vi "wavelenght and intensity New.vi"(8 "Command":string, 10 "Number of Fiber":string, 11 "VISA resource name":string) -> (0 "LED":bool, 1 "LED COLOR":string, 2 "INTENSITY":i32, 3 "WAVELENGHT":dbl)   [LabVIEW 2023]
panel:
  out "number_LED":i32
  out "Blue":u8
  out "Green":u8
  out "Red":u8
  out "VISA resource name":refnum<visa-resource-name>="ASRL34::INSTR"
  out "OUTPUT":string
  # "NOTE: remember plug-in the LED Analyser\ncable before run this VI and to select the\nVISA resource name (port)"
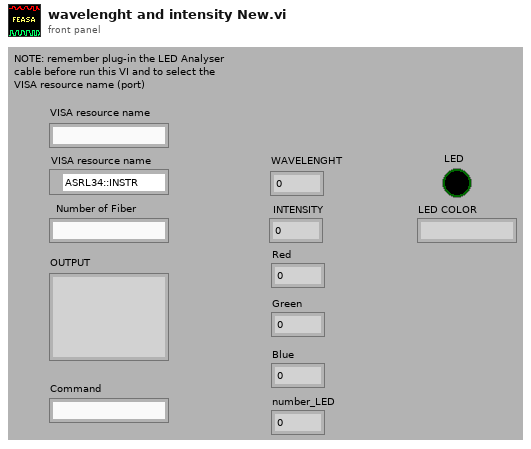
[diagram p1: front panel]
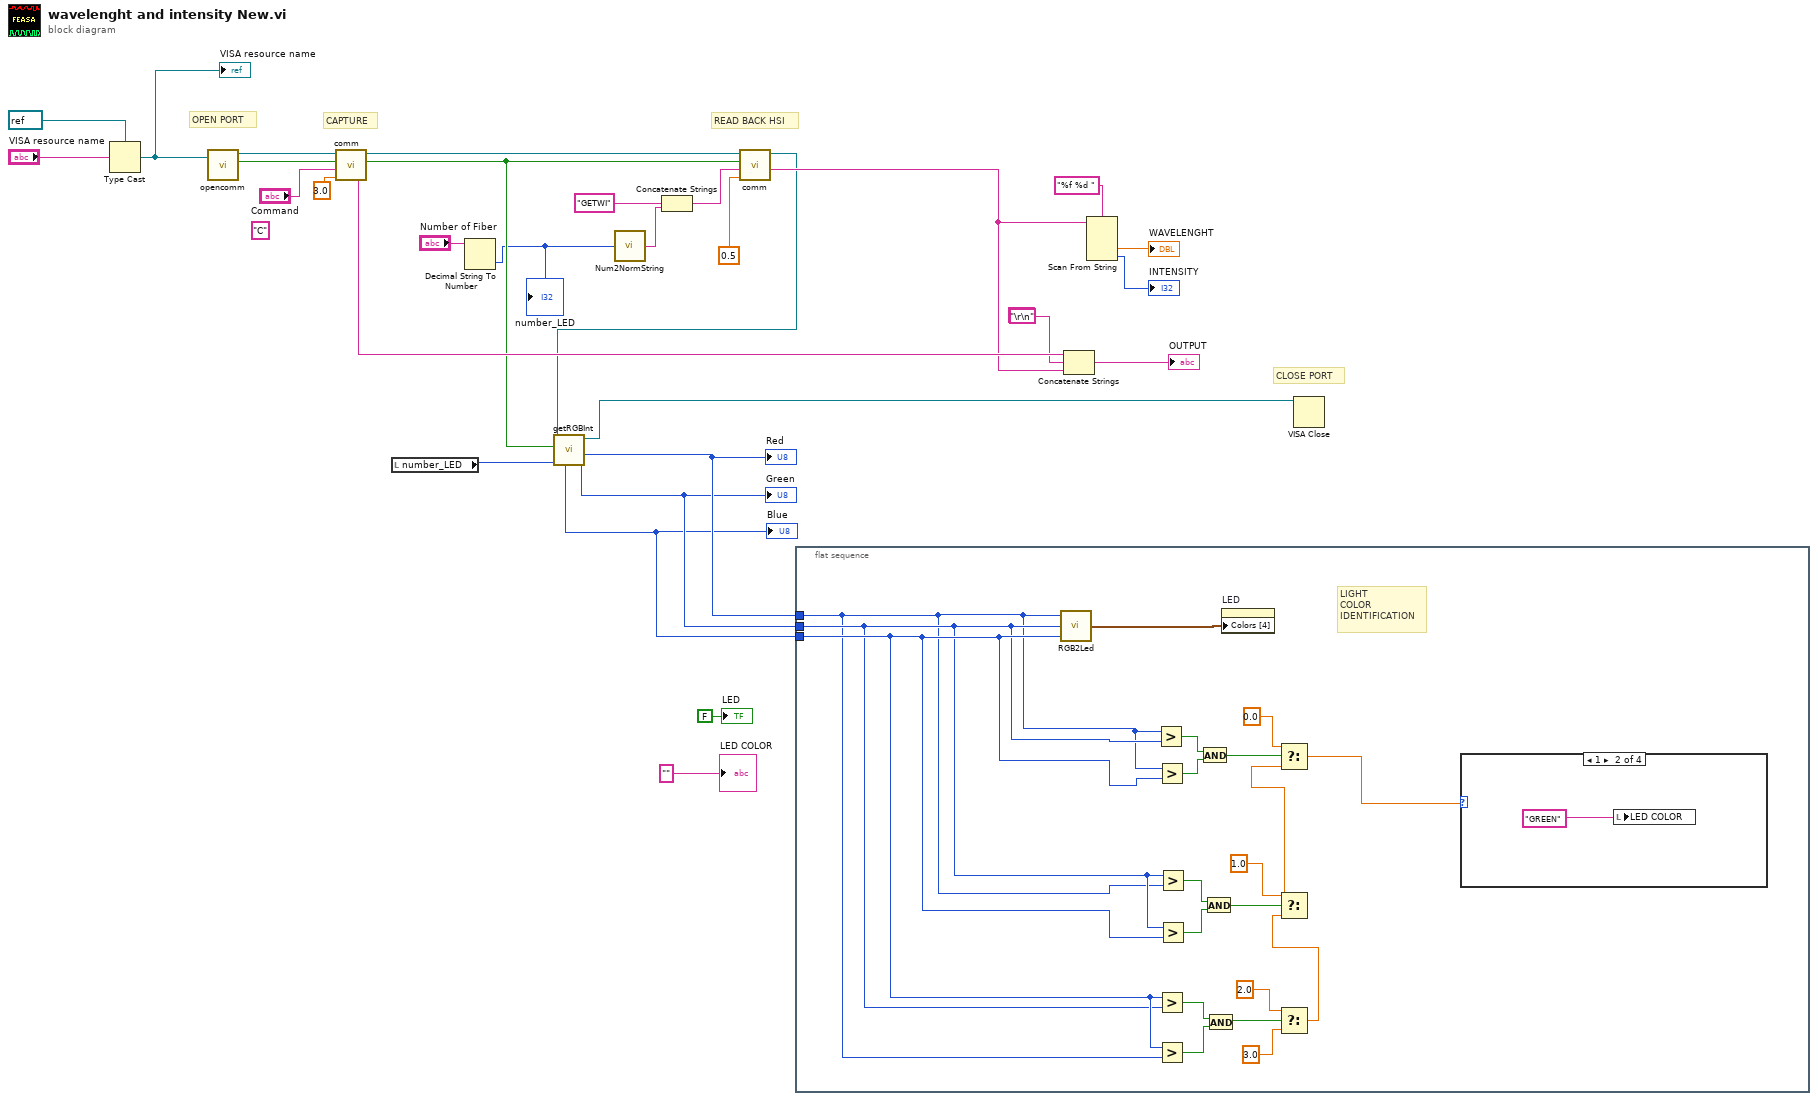
[diagram p0: block diagram]
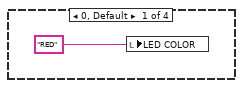
[diagram p2: hidden frame]
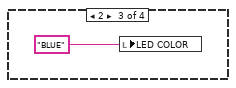
[diagram p3: hidden frame]
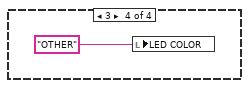
[diagram p4: hidden frame]
diagram:
  (unwired) "\r\n"
  (unwired) "C" ("Command")
  # "CLOSE PORT"
  # "READ BACK HSI"
  # "CAPTURE"
  # "OPEN PORT"
  n1 = Type Cast(type=refnum<visa-resource-name> refnum ("VISA resource name"), x="VISA resource name") -> (*(type *) &x=w3:refnum<visa-resource-name>)
  "VISA resource name" <- w3
  n2 = call "opencomm.vi"("VISA resource name"=w3) -> ("duplicate VISA resource name"=w30:refnum<visa-resource-name>, "Error"=w29:bool)  [unwired: 3 in]
  n3 = call "comm.vi"("Timeout (s)"=3.0, "Command"="Command", "Error"=w29, "VISA resource name"=w30) -> ("Response"=w23:string, "Error"=w15:bool, "dup VISA resource name"=w16:refnum<visa-resource-name>)  [unwired: 2 in, 1 out]
  n4 = local read "number_LED"() -> (w14:i32)
  n5 = Decimal String To Number(string="Number of Fiber") -> (number=w2:i32)  [unwired: 2 in, 1 out]
  "number_LED" <- w2
  n6 = call "Num2NormString.vi"("Number"=w2) -> ("Normalized String Number"=w27:string)
  n7 = Concatenate Strings("GETWI" ("Command"), w27) -> (w26:string)
  n8 = call "comm.vi"("Timeout (s)"=0.5, "Command"=w26, "Error"=w15, "VISA resource name"=w16) -> ("Response"=w20:string, "dup VISA resource name"=w13:refnum<visa-resource-name>)  [unwired: 2 in, 2 out]
  n9 = call "getRGBInt.vi"("Fiber Num"=w14, "Error"=w15, "VISA resource name"=w13) -> ("Green"=w10:u8, "Red"=w11:u8, "dup VISA resource name"=w12:refnum<visa-resource-name>, "Blue"=w9:u8)  [unwired: 3 in, 2 out]
  "Red" <- w11
  "Green" <- w10
  "Blue" <- w9
  n10 = flat-sequence {
    tunnel: w11 -> [w47]
    tunnel: w10 -> [w48]
    tunnel: w9 -> [w49]
    frame #0 {
      # "LIGHT\nCOLOR\nIDENTIFICATION"
      n11 = call "RGB2Led.vi"("B"=w49, "G"=w48, "R"=w47) -> ("Colors [4]"=w50:cluster{u32, u32}[])
      n12 = Greater?(x=w47, y=w48) -> (0:w46:bool)
      n13 = Greater?(x=w47, y=w49) -> (0:w45:bool)
      n14 = Greater?(x=w49, y=w48) -> (0:w42:bool)
      n15 = Greater?(x=w49, y=w47) -> (0:w41:bool)
      n16 = Greater?(x=w48, y=w47) -> (0:w44:bool)
      n17 = Greater?(x=w48, y=w49) -> (0:w43:bool)
      n18 = And(x=w46, y=w45) -> (x .and. y?=w40:bool)
      n19 = And(x=w44, y=w43) -> (x .and. y?=w37:bool)
      n20 = And(x=w42, y=w41) -> (x .and. y?=w34:bool)
      n21 = property on="LED" class="Bool (strict)"("Colors [4]"=w50) -> ()  [unwired: 2 in, 2 out]
      n22 = Select(t=2.0, s=w34, f=3.0) -> (s? t:f=w31:dbl)
      n23 = Select(t=1.0, s=w37, f=w31) -> (s? t:f=w35:dbl)
      n24 = Select(t=0.0, s=w40, f=w35) -> (s? t:f=w38:dbl)
      n25 = case shown="1" w38 {
        frame 0, Default {
          n26 = local write "LED COLOR"("RED") -> ()
        }
        frame 1 {
          n27 = local write "LED COLOR"("GREEN") -> ()
        }
        frame 2 {
          n28 = local write "LED COLOR"("BLUE" ("LED COLOR")) -> ()
        }
        frame 3 {
          n29 = local write "LED COLOR"("OTHER" ("LED COLOR")) -> ()
        }
      }
    }
  }
  n30 = Concatenate Strings(w23, "\r\n", w20) -> (→"OUTPUT":string)
  n31 = Scan From String(format string="%f %d ", input string=w20) -> (output 1=→"WAVELENGHT":dbl, output 2=→"INTENSITY":i32)  [unwired: 4 in, 3 out]
  n32 = VISA Close(VISA resource name=w12) -> ()  [unwired: 1 in, 1 out]
  "LED" <- FALSE ("LED")
  "LED COLOR" <- "" ("LED COLOR")
